vi "Untitled 4.vi"() -> ()   [LabVIEW 2013]
uses:
  <vilib>/addons/control/pid/pid.llb/PID (DBL).vi
  <vilib>/addons/control/pid/NI_PID_pid.lvlib
panel:
  out "Waveform Chart 2":dbl(graph)
  out "Waveform Chart":dbl(graph)
  in  "stop":bool
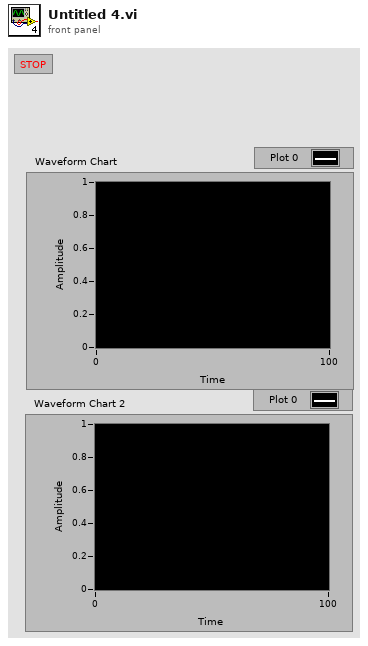
[diagram p1: front panel]
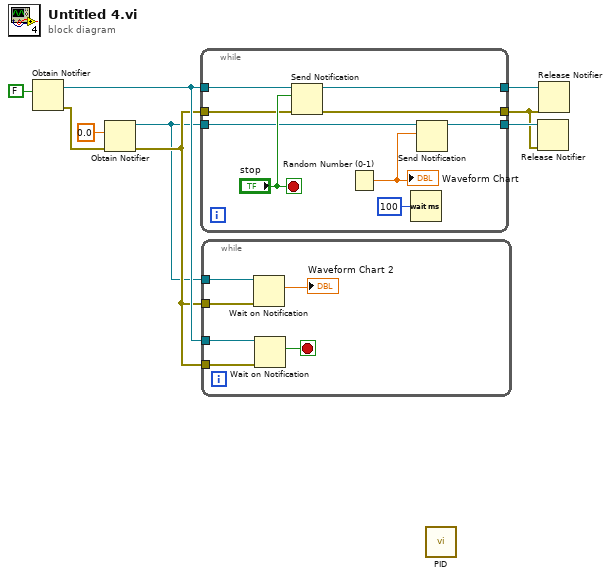
[diagram p0: block diagram]
diagram:
  n1 = Obtain Notifier(notification data type=FALSE) -> (notifier out=w5:refnum<notifier>, error out=w9:errorcluster)  [unwired: 3 in, 1 out]
  n2 = Obtain Notifier(notification data type=0.0 ("element data type"), error in (no error)=w9) -> (notifier out=w1:refnum<notifier>, error out=w2:errorcluster)  [unwired: 2 in, 1 out]
  n3 = while {
    tunnel: w5 -> [w18]
    tunnel: [w16] -> w6
    tunnel: w2 -> [w15]
    tunnel: [w12] -> w4
    tunnel: w1 -> [w13]
    tunnel: [w14] -> w3
    stop <- "stop" stop-if-true
    n4 = Send Notification(notification="stop", notifier=w18, error in (no error)=w15) -> (notifier out=w16:refnum<notifier>, error out=w14:errorcluster)
    n5 = Random Number (0-1)() -> (number: 0 to 1=w11:dbl)
    "Waveform Chart" <- w11
    n6 = Wait (ms)(milliseconds to wait=u32 100) -> ()  [unwired: 1 out]
    n7 = Send Notification(notification=w11, notifier=w13) -> (notifier out=w12:refnum<notifier>)  [unwired: 1 in, 1 out]
  }
  n8 = while {
    tunnel: w5 -> [w23]
    tunnel: w2 -> [w22]
    tunnel: w2 -> [w21]
    tunnel: w1 -> [w20]
    stop <- w24 stop-if-true
    n9 = Wait on Notification(notifier=w20, error in (no error)=w21) -> (notification=→"Waveform Chart 2":dbl)  [unwired: 2 in, 3 out]
    n10 = Wait on Notification(notifier=w23, error in (no error)=w22) -> (notification=w24:bool)  [unwired: 2 in, 3 out]
  }
  n11 = call-poly <vilib>:"PID.vi"() -> ()  [unwired: 10 in, 2 out]
  n12 = Release Notifier(notifier=w4, error in (no error)=w3) -> ()  [unwired: 1 in, 3 out]
  n13 = Release Notifier(notifier=w6, error in (no error)=w3) -> ()  [unwired: 1 in, 3 out]
